vi "Clean up Phasor Parameters String.vi"(8 "Error In":errorcluster, 10 "Cluster Label":string, 11 "String in":string) -> (0 "Error Out":errorcluster, 3 "String out":string)   [LabVIEW 2019]
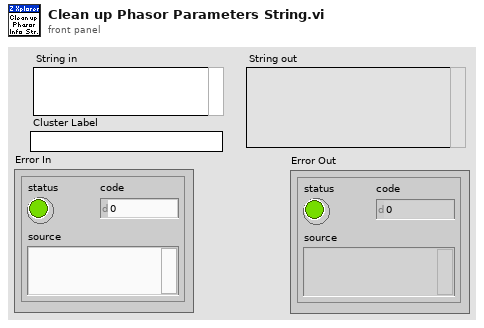
[diagram p1: front panel]
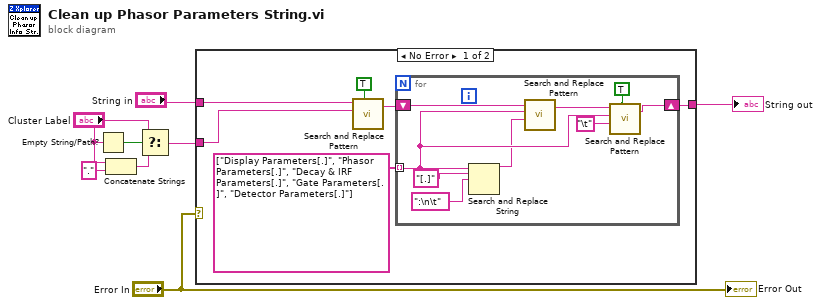
[diagram p0: block diagram]
diagram:
  n1 = Empty String/Path?(string/path="Cluster Label") -> (empty?=w5:bool)
  n2 = Concatenate Strings("Cluster Label", "." ("string")) -> (w1:string)
  n3 = Select(t="Cluster Label", s=w5, f=w1) -> (s? t:f=w4:string)
  n4 = case shown="No Error" "Error In" {
    tunnel: "String in" -> [w9 w24]
    tunnel: w4 -> [w10 _]
    tunnel: [w11 w24] -> w7
    frame No Error {
      n5 = call <vilib>:"Search and Replace Pattern.vi"("string"=w9, "regular expression (\"\")"=w10, "replace all? (F)"=TRUE) -> ("result string"=w12:string)  [unwired: 2 in, 1 out]
      n6 = for {
        tunnel: string[] ["Display Parameters[.]", "Phasor Parameters[.]", "Decay & IRF Parameters[.]", "Gate Parameters[.]", "Detector Parameters[.]"] ("regular expression (\"\")") -> [w18] mode=indexing
        shift-right: [w20] -> w11
        shift-left: w12 -> [w23]
        n7 = Search and Replace String(input string=w18, search string="[.]" ("regular expression (\"\")"), replace string=":\n\t" ("replace string (\"\")")) -> (result string=w15:string)  [unwired: 5 in, 3 out]
        n8 = call <vilib>:"Search and Replace Pattern.vi"("string"=w23, "regular expression (\"\")"=w18, "replace string (\"\")"=w15) -> ("result string"=w22:string)  [unwired: 2 in, 1 out]
        n9 = call <vilib>:"Search and Replace Pattern.vi"("string"=w22, "regular expression (\"\")"=w18, "replace string (\"\")"="\t", "replace all? (F)"=TRUE) -> ("result string"=w20:string)  [unwired: 1 in, 1 out]
      }
    }
    frame Error {
    }
  }
  "String out" <- w7
  "Error Out" <- "Error In"
